vi "Ke2000 Current Config Setup.vi"(7 "Current Config":enum16{"DCI", "ACI"}(ring), 8 "error in (no error)":errorcluster, 10 "Auto Range(T/F)":bool, 11 "VISA resource name":refnum<visa-resource-name>) -> (0 "error out":errorcluster, 3 "VISA resource name out":refnum<visa-resource-name>)   [LabVIEW 2012]
doc: "This VI is a Current Config\nDC current is by default\nAuto Range is OFF"
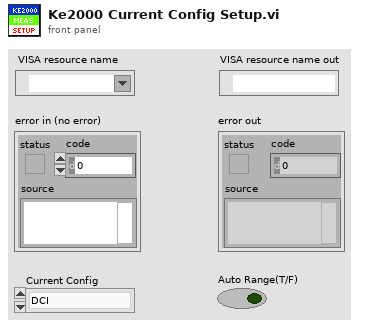
[diagram p1: front panel]
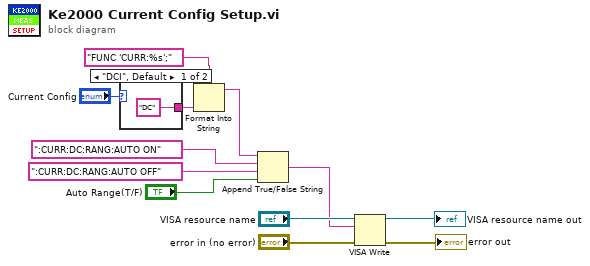
[diagram p0: block diagram]
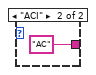
[diagram p2: hidden frame]
diagram:
  n1 = case shown="\"DCI\", Default" "Current Config" {
    tunnel: ["DC" ("format string") "AC" ("format string")] -> w2
    frame "DCI", Default {
    }
    frame "ACI" {
    }
  }
  n2 = Format Into String(format string="FUNC 'CURR:%s';", w2) -> (resulting string=w8:string)  [unwired: 2 in, 1 out]
  n3 = Append True/False String(1:"Auto Range(T/F)", 2:":CURR:DC:RANG:AUTO OFF" ("true string"), 3:":CURR:DC:RANG:AUTO ON" ("true string"), 4:w8) -> (0:w4:string)
  n4 = VISA Write(VISA resource name="VISA resource name", write buffer=w4, error in (no error)="error in (no error)") -> (VISA resource name out=→"VISA resource name out":refnum<visa-resource-name>, error out=→"error out":errorcluster)  [unwired: 1 out]
